vi "Volume data viewer tool.vi"() -> ()   [LabVIEW 2020]
uses:
  <vilib>/addons/Biomedical/NI_BMTK_Controls.lvlib
  <vilib>/addons/Biomedical/Controls/Medical Image/Medical Image 2D Viewer Helper (2D U16).vi
  Typedefs/Save-Load enum.ctl
  <vilib>/addons/Biomedical/Controls/Medical Image/2D Image Viewer/Medical Image 2D Viewer.xctl
panel:
  out "2D Viewer":i32[][][](xcontrol)
  in  "Selected Plane":i32(slide) scale=1.0..5.0
  in  "TDMS file path & name":path=path "C:/Users/Theo/Desktop/Volume Acquisition/Volume acquisition TDMS data files/001.tdms"
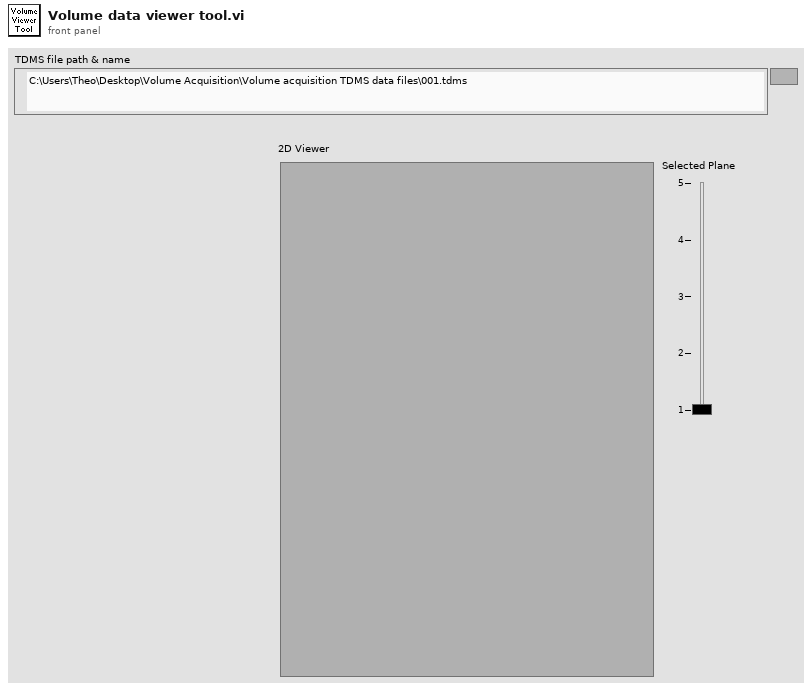
[diagram p1: front panel]
types:
  T1 = typedef "Save-Load enum.ctl" = enum16{"Save to file", "Load from file", "Compare from file", "Save Backup"}
  T2 = typedef "Header parameters cluster-ALL.ctl" = cluster{"LOGIN":T3, "GLOBAL PARAMETERS":T4, "IMAGING MODES":T6, "TIME SERIES":T7, "MOTOR Z-STACK ":T10, "AOL Z-STACK":T11, "FUNCTIONAL IMAGING":T12, "VOLUME IMAGING":T12, "MOVEMENT CORRECTION":T16, "CALIBRATION":T18, "STATISTICS":T19, "BIOLOGY INFORMATION":T20, "Calibration Data":T21}
  T3 = typedef "Header params -Login.ctl" = cluster{"User":string, "Profile":string, "Software Version":string, "Experiment Date Time":timestamp}
  T4 = typedef "Header params-Global Parameters.ctl" = cluster{"MicroscopeID":string, "Microscope Type":string, "Objective":string, "Field of View (um)":dbl, "Fill time (us)":dbl, "Experiment Type":T5, "Stimuli Trigger":bool, "Speed Logging":bool}
  T5 = typedef "Experiment Type.ctl" = enum16{"In vivo", "In vitro", "Testing", "Calibration", "Other"}
  T6 = typedef "Header params-Imaging Modes.ctl" = cluster{"Time Series":bool, "Motor Zstack":bool, "AOL Zstack":bool, "Functional Imaging":bool, "Volume Imaging":bool}
  T7 = typedef "Header params-Time Series.ctl" = cluster{"Basic Image meta data":T8, "AOL z":dbl}
  T8 = typedef "Header params-Basic image meta data.ctl" = cluster{"Wavelength (nm)":dbl, "# averaged frames":dbl, "laser power (%)":dbl, "Pockels":dbl, "pixel dwell time (us)":dbl, "pmt 1":dbl, "pmt 2":dbl, "back apperture":dbl, "zoom":dbl, "field of view":dbl, "Frame Size":T9, "AOL x centre":dbl, "AOL y centre":dbl, "Stage x position":dbl, "Stage y position":dbl, "Stage z position":dbl}
  T9 = typedef "Frame Size.ctl" = u16
  T10 = typedef "Header params-Motor Z-stack.ctl" = cluster{"Hdr Basic Image meta data":T8, "Z Start":dbl, "Z Stop":dbl, "No of Planes":i32, "Laser Power (%) at Z Start":dbl, "Laser Power (%) at Z Stop":dbl}
  T11 = typedef "Header params-AOL Z-stack.ctl" = cluster{"Hdr Basic Image meta data":T8, "Z Start":dbl, "Z Stop":dbl, "No of Planes":i32, "Laser Power (%) at Z Start":dbl, "Laser Power (%) at Z Stop":dbl}
  T12 = typedef "Header params-Functional Imaging.ctl" = cluster{"Functional Mode":T13, "Variable Length":bool, "Variable Resolution":bool, "Pockels Modulation":bool, "Stimuli Trigger":bool, "Cool down enabled":bool, "AOL Mode":T14, "Plane Mode":T15, "Miniscan Dwell time per pixel (us)":dbl, "poi dwell time":dbl, "Number of trials":dbl, "Number of cycles":dbl, "Number of pois":dbl, "Number of miniscans":dbl, "Number of pixels in miniscan":dbl, "Rectangle ROI length":dbl, "Rectangle ROI height":dbl, "Frame rate (fps)":dbl, "Acquisition Length":dbl, "video length (sec)":dbl, "Stimuli delay (sec)":dbl, "Cool down time (sec)":dbl, "Basic Image meta data":T8, "Z Start (um)":dbl, "Z Stop (um)":dbl}
  T13 = typedef "Functional Mode.ctl" = enum16{"Point", "Line", "Patch", "Plane", "Volume"}
  T14 = typedef "AOL modes.ctl" = enum16{"Raster", "Structural", "Pointing", "Mini Scan", "Alignment"}
  T15 = typedef "Plane Mode.ctl" = u16
  T16 = typedef "Header params-Movement correction.ctl" = cluster{"Movement Correction":bool, "Axial Reference":bool, "Reference Source":T17, "Full Frame Size":dbl, "Reference Field of View":dbl, "Reference Zoom":dbl, "Reference dwell time (us)":dbl, "Reference X Pixels":dbl, "Reference Y Pixels":dbl, "Number of Z lines":dbl, "Size of Z pixels":dbl, "Axial Pixels":dbl, "Ignore Z lines":dbl, "Reference Scan Cycles":dbl, "Reference Threshold XY":dbl, "Reference Threshold Z":dbl, "Reference Average XY":dbl, "Reference Average Z":dbl, "Proportional Scale":dbl, "Integral Scale":dbl, "Proportional Scale Z":dbl, "Integral Scale Z":dbl, "Diff Threshold":dbl, "Diff Threshold Z":dbl, "Sliding Average":bool, "Reference count reset enabled":bool, "Scan Interval (ms)":dbl, "Ref Plot Refresh Rate (ms)":dbl}
  T17 = typedef "Reference source.ctl" = enum16{"Green channel", "Red channel"}
  T18 = typedef "Header params-Calibration Setup.ctl" = cluster{"Pockels Calibration File":path, "Calibration_ini file":path, "Setup_ini file":path}
  T19 = typedef "Header params-statistics.ctl" = cluster{"Z-stack duration (sec)":dbl, "Number of acquired data-points":dbl, "Acquisition time (ms)":dbl, "Number of acquired frames":dbl, "Intertrial times":dbl[]}
  T20 = typedef "Biology Information.ctl" = cluster{"Animal Code or Name":string, "Animal DoB":string, "Animal Age":string, "Animal Sex":string, "Animal Weight":string, "Date of Injection":string, "Date of Implant":string, "Site of Injection":string, "Animal Ear Notch":string, "AAV constructs":string, "Genetic background":string, "Optical reporter":string, "Region of brain imaged":string, "Other \ncomments":string}
  T21 = typedef "Header params-calibration data.ctl" = cluster{"Objective Name":string, "Calibration Wavelength":dbl, "Sum X":dbl, "Sum Y":dbl, "Diff X":dbl, "Diff Y":dbl, "Distortion Correction":dbl, " Z norm to um Scaling":dbl, " X norm to um Scaling":dbl}
  T22 = cluster{"Number of cycles":i32, "number of planes":i32, "number of miniscans in a Plane":i32, "number of pixels in a miniscan":i32}
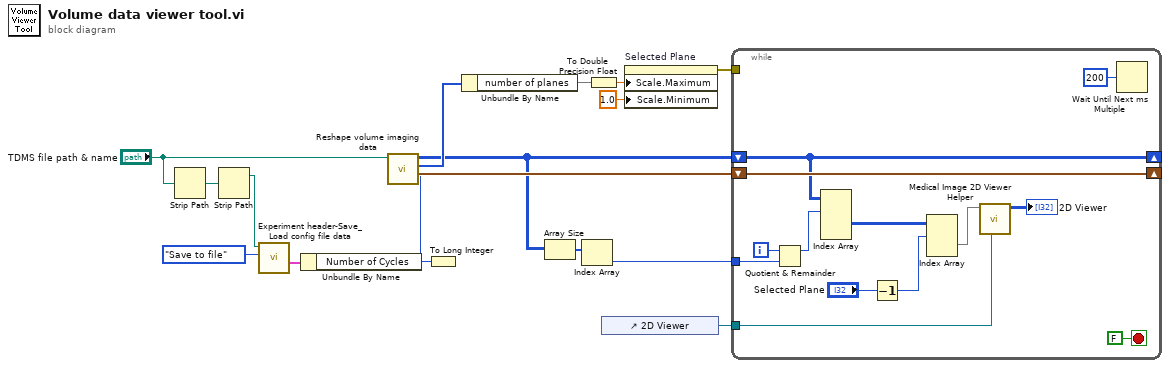
[diagram p0: block diagram]
diagram:
  n1 = Strip Path(path="TDMS file path & name") -> (stripped path=w5:path)  [unwired: 1 out]
  n2 = Strip Path(path=w5) -> (stripped path=w3:path)  [unwired: 1 out]
  n3 = call "Experiment header-Save_Load config file data.vi"(10:Save-Load_enum."Save to file" ("Function"), "Experiment data folder path"=w3) -> ("All header parameters out"=w6:T2)  [unwired: 8 in, 1 out]
  n4 = Unbundle By Name(w6) -> ("Number of Cycles"=w2:u64)
  n5 = To Long Integer(number=w2) -> (32bit integer=w1:i32)
  n6 = call "Reshape volume imaging data.vi"(9:w1, "TDMS file path & name"="TDMS file path & name") -> ("Volumetric parameters"=w9:T22, "Single channel data"=w10:u16[], "Channel 4D data"=w8:u16[][][][])  [unwired: 4 in, 3 out]
  n7 = Unbundle By Name(w10) -> ("number of planes"=w15)
  n8 = Array Size(array=w8) -> (size(s)=w17:i32[])
  n9 = Index Array(array=w17) -> (element=w16:i32)  [unwired: 1 in]
  n10 = To Double Precision Float(number=w15) -> (double precision float=w11:dbl)
  n11 = control-ref of="2D Viewer"() -> (w13:refnum<vi>)
  n12 = property on="Selected Plane" class="Slide (strict)"("Scale.Maximum"=w11, "Scale.Minimum"=1.0 ("Scale.Range:Minimum")) -> (error out=w12:errorcluster)  [unwired: 2 in, 1 out]
  n13 = while {
    shift-right: [w25] -> _
    shift-left: w8 -> [w25]
    shift-right: [w28] -> _
    shift-left: w9 -> [w28]
    tunnel: w16 -> [w27]
    tunnel: w13 -> [w19]
    tunnel: w12 -> [_]
    i -> [w26]
    stop <- FALSE stop-if-true
    n14 = Quotient & Remainder(x=w26, y=w27) -> (x-y*floor(x/y)=w24:i32)  [unwired: 1 out]
    n15 = Index Array(array=w25, index (dim 0)=w24) -> (element=w20:u16[][][])  [unwired: 3 in]
    n16 = Decrement(x="Selected Plane") -> (x-1=w22:i32)
    n17 = Index Array(array=w20, index (dim 0)=w22) -> (element=w18:u16[][])  [unwired: 2 in]
    n18 = call-poly <vilib>:"Medical Image 2D Viewer Helper.vi"("2D Viewer"=w19, "2D array in"=w18) -> ("3D array out"=→"2D Viewer":i32[][][])  [unwired: 8 in, 1 out]
    n19 = Wait Until Next ms Multiple(millisecond multiple=u32 200) -> ()  [unwired: 1 out]
  }
